vi "Register State as Status Example.vi"() -> ()   [LabVIEW 2017, in "Register State as Status Example.lvlib"]
uses:
  Register State as Status Example.lvlib
  user.lib/_NEVSTOP/Communicable State Machine(CSM)/Utility/_support/Periodic String Filter Level.ctl
  user.lib/_NEVSTOP/Communicable State Machine(CSM)/_Support/Common/Format Timestamp.vi
  user.lib/_NEVSTOP/Communicable State Machine(CSM)/AdvanceAPI/CSM - Revert Arguments-Safe String.vi
  user.lib/_NEVSTOP/Communicable State Machine(CSM)/AdvanceAPI/CSM - Make String Arguments Safe.vi
  user.lib/_NEVSTOP/Communicable State Machine(CSM)/AdvanceAPI/CSM - Break Down Multiple States String.vi
  user.lib/_NEVSTOP/Communicable State Machine(CSM)/AdvanceAPI/CSM - Compact Multiple States.vi
  user.lib/_NEVSTOP/Communicable State Machine(CSM)/AdvanceAPI/CSM - Keywords.vi
  user.lib/_NEVSTOP/Communicable State Machine(CSM)/_Shared/Trim Single-line Text.vi
  user.lib/_NEVSTOP/Communicable State Machine(CSM)/Communicable State Machine.lvlib
  user.lib/_NEVSTOP/Communicable State Machine(CSM)/Utility/Periodic String Filter Setting.ctl
  user.lib/_NEVSTOP/Communicable State Machine(CSM)/_Shared/CSM Shared.lvlib
panel:
  in  "Macro: Exit -> submodule2":bool
  in  "Macro: Exit -@submodule1":bool
  out "LogInQ":i32
  out "State History":string
  out "log handling Speed(#/s)":dbl
  out "LogInQ change(#/s)":dbl
  out "Level":T1
  in  "Registration":string="Macro: Initialize@* >> Echo: Echo1 -><register> \nAPI: API1@* >> Echo: Echo1-><register>\nAPI: API2@SubModule1 >> Echo: Echo2 -><register>\nEcho: Echo2@main >> API: API1@submodule1 -><register>\nExit@submodule1 >> Echo: Echo1 -><register>\nMacro: Exit@submodule2 >> Echo: Echo1 -><register>"
  in  "API: API2 -> submodule2":bool
  in  "API: API1 -> submodule2":bool
  in  "API: API2 -@submodule1":bool
  in  "API: API1 -@submodule1":bool
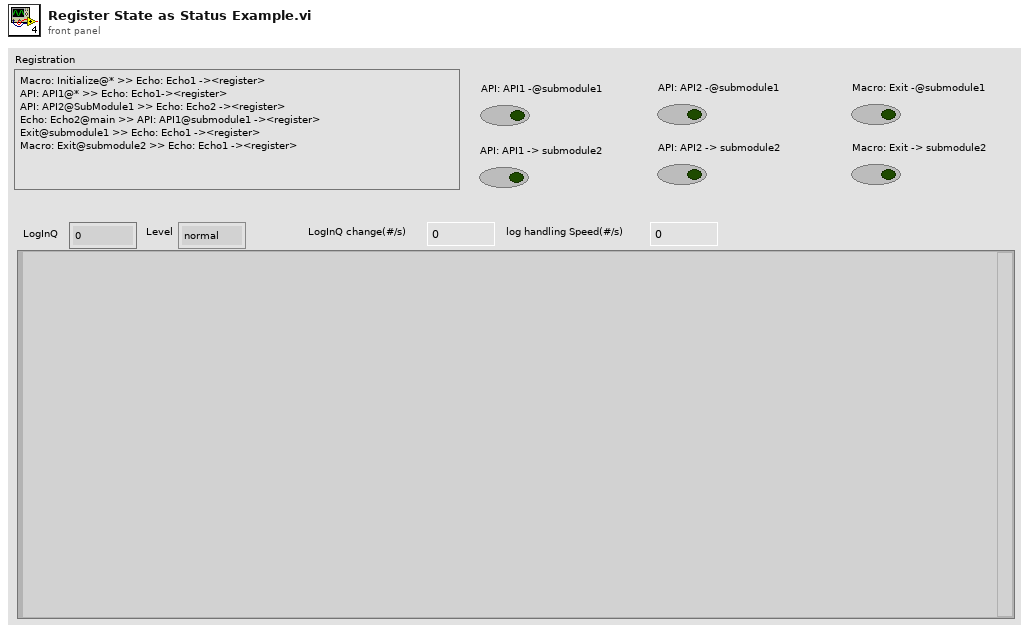
[diagram p1: front panel]
types:
  T1 = typedef "Communicable State Machine.lvlib/Periodic String Filter Level.ctl" = enum16{"normal", "L1", "L2", "L3", "L4"}
  T2 = enum32{"Invalid", "Standard", "Closed", "Hidden", "Minimized", "Maximized"}
  T3 = enum32{"invalid app kind", "Development System", "Run Time System", "Student Edition", "Embedded LabVIEW", "Evaluation", "Custom"}
  T4 = typedef "Communicable State Machine.lvlib/_CSM_Response Source Message.ctl" = cluster{"‘State":string, "’Arguments":string, "’Error":errorcluster}
  T5 = cluster{"Current VI Reference":refnum<vi>, "Close Panel on Exit?":bool}
  T6 = cluster{"Core":cluster{"Current VI Reference":refnum<vi>, "Close Panel on Exit?":bool}, "Your Boolean data":bool, "Your string data":string}
  T7 = typedef "Communicable State Machine.lvlib/_CSM_STATE_CALL_REASON.ctl" = enum16{"LocalCall", "RemoteCall", "StatusCallback"}
  T8 = typedef "Communicable State Machine.lvlib/Periodic String Filter Setting.ctl" = cluster{"threashold(#/s)":dbl, "Check Peroid(s)":dbl}
  T9 = typedef "Communicable State Machine.lvlib/_CSM_GlobalLog_MSG.ctl" = cluster{"Name (\"\" to Use UUID)":string, "Current State":string, "Arguments":string, "Source Message":T4, "Source Module":string, "Complete(T)/Start(F)":bool, "LogType":T10, "Time Stamp":timestamp}
  T10 = typedef "Communicable State Machine.lvlib/_CSM_GlobalLog_MSG_TYPE.ctl" = enum16{"User Log", "State Change", "Status", "Interrupt", "Register", "Unregister", "Error Log", "Module Created", "Module Destroyed"}
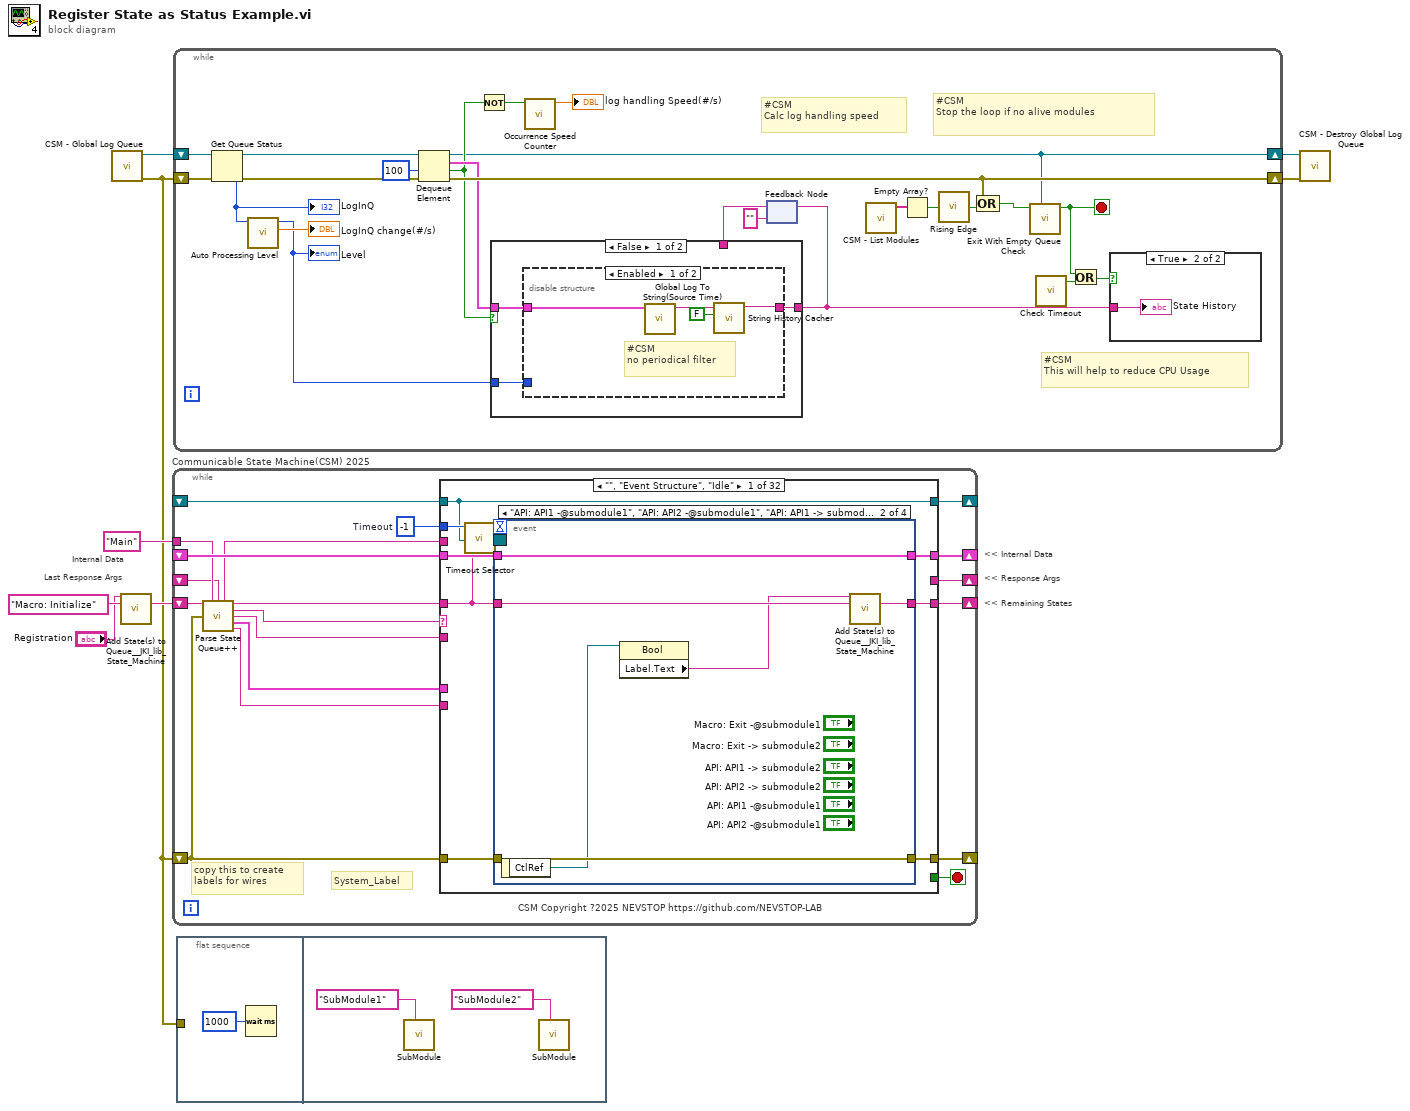
[diagram p0: block diagram]
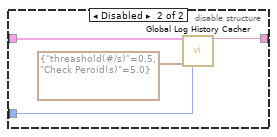
[diagram p2: hidden frame]
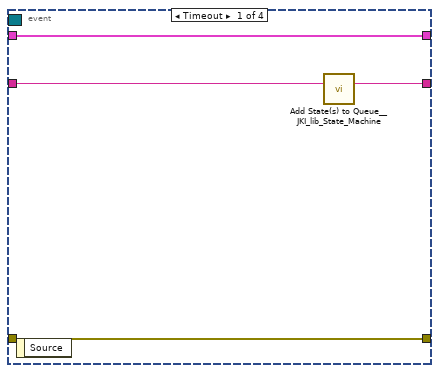
[diagram p5: hidden frame]
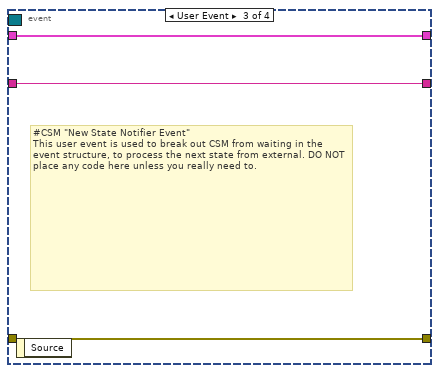
[diagram p6: hidden frame]
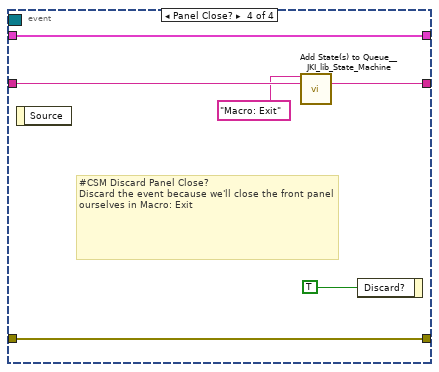
[diagram p7: hidden frame]
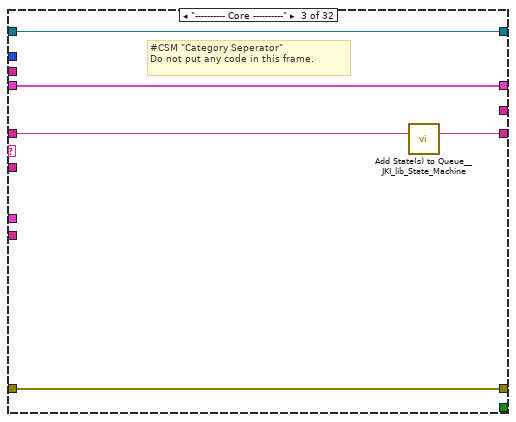
[diagram p9: hidden frame]
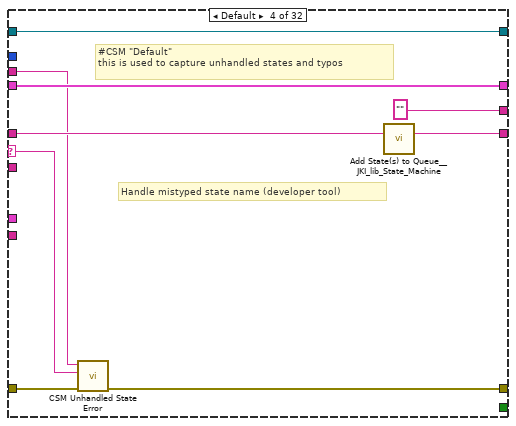
[diagram p10: hidden frame]
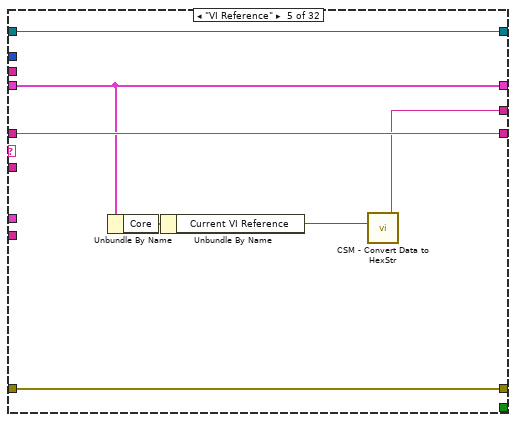
[diagram p11: hidden frame]
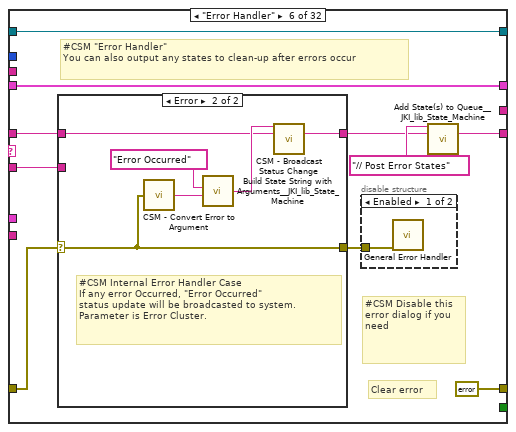
[diagram p12: hidden frame]
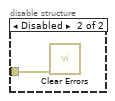
[diagram p13: hidden frame]
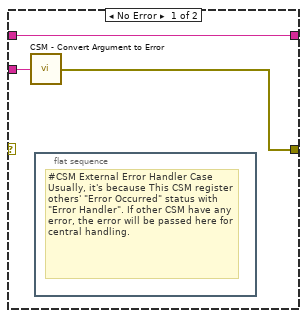
[diagram p14: hidden frame]
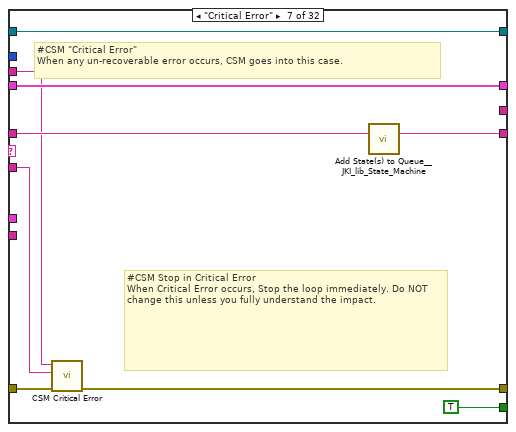
[diagram p15: hidden frame]
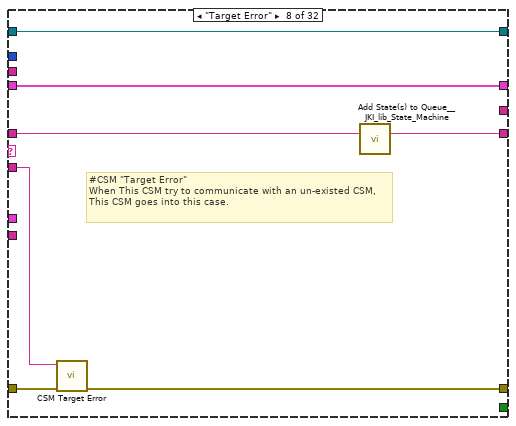
[diagram p16: hidden frame]
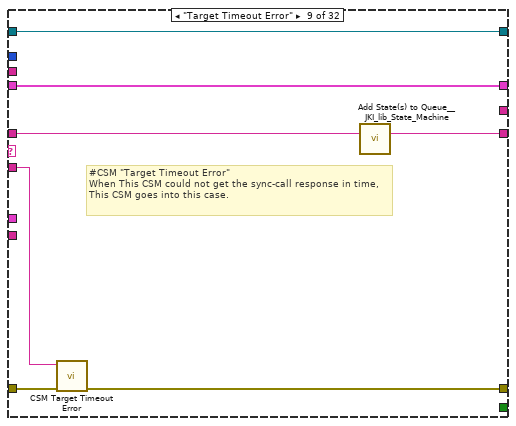
[diagram p17: hidden frame]
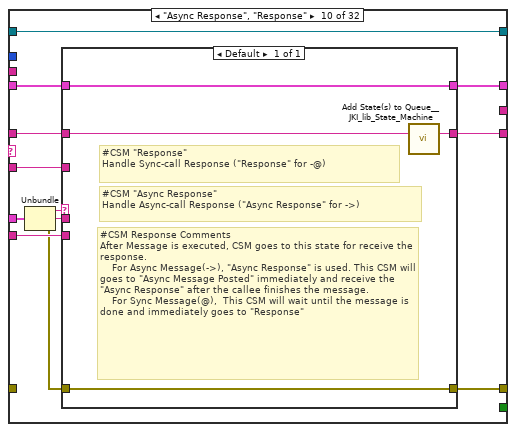
[diagram p18: hidden frame]
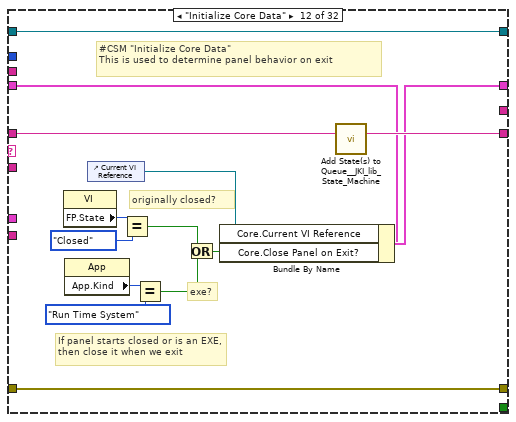
[diagram p20: hidden frame]
diagram:
  # "Last Response Args"
  # "Internal Data"
  # "<< Internal Data"
  # "<< Response Args"
  # "<< Remaining States"
  n1 = call "CSM - Global Log Queue.vi"() -> ("error out"=w1:errorcluster, "GlobalEvent Queue"=w2:refnum<queue>)  [unwired: 10 in]
  n2 = call <vilib>:"Add State(s) to Queue__JKI_lib_State_Machine.vi"("State(s) in Front (\"\")"="Registration", "State(s) in (\"\")"="Macro: Initialize" ("Init State(\"Macro: Initialize\")")) -> ("States Out"=w8:string)  [unwired: 13 in]
  n3 = while "Communicable State Machine(CSM) 2025" {
    shift-right: [w22] -> _
    shift-left: _ -> [w21]
    shift-right: [w25] -> _
    shift-left: w1 -> [w19]
    shift-right: [w24] -> _
    shift-left: w8 -> [w26]
    tunnel: "Main" ("Name(\"\" to use uuid)") -> [w15]
    shift-right: [w18] -> _
    shift-left: _ -> [w9]
    shift-right: [w17] -> _
    shift-left: _ -> [w16]
    stop <- w23 stop-if-true
    w20 = -1  # Timeout
    # "copy this to create labels for wires"
    # "System_Label"
    # "CSM Copyright ?2025 NEVSTOP https://github.com/NEVSTOP-LAB"
    n4 = call "Parse State Queue++.vi"("State Queue"=w26, "Name (\"\" to Use UUID)"=w15, "Response Arguments"=w9, "Previous Error"=w19) -> ("Name Used"=w10:string, "Remaining States"=w27:string, "Current State"=w14:string, "Arguments"=w13:string, ">> Response Source Message >>"=w12:T4, ">> Source CSM >>"=w11:string)  [unwired: 6 in]
    n5 = case shown="\"\", \"Event Structure\", \"Idle\"" w14 {
      selector: w14 -> [_ _ _ w67 _ _ _ _ _ _ _ _ _ _ _ _ _ _ _ _ _ _ _ _ _ _ _ _ _ _ _ _]
      tunnel: w27 -> [w28 w58 w64 w72 w79 w85 w108 w114 w121 w130 w143 w158 w164 w169 w177 w184 w189 w196 w200 w206 w211 w218 w234 w304 w310 w323 w326 w331 w337 w345 w355 w370]
      tunnel: w13 -> [_ _ _ _ _ w84 w103 w113 w120 w129 _ _ _ _ _ _ _ _ _ _ _ w213 w228 _ _ _ _ _ w334 _ w350 _]
      tunnel: w21 -> [w35 w57 w61 w70 w78 w89 w109 w116 w123 w132 w142 w151 w162 w166 _ w179 w186 w195 w199 w203 w209 w216 w230 w301 w307 w320 w325 w330 w336 w342 w352 w367]
      tunnel: [w34 w59 w62 w65 w80 errorcluster {"status"=FALSE, "code"=0, "source"=""} ("error out") w104 w111 w118 w135 w144 w155 w161 w167 w174 w180 w187 w190 w198 w204 w208 w214 w231 w302 w308 w321 w327 w332 w338 w343 w353 w368] -> w25
      tunnel: w19 -> [w33 w59 w62 w73 w80 w86 w110 w112 w119 _ w144 w155 w161 w167 w174 w181 w187 _ w201 w204 w208 w215 w232 w302 w308 w321 w327 w332 w338 w343 w353 w368]
      tunnel: [w36 w58 w63 w71 w79 w81 w107 w117 w124 w131 w143 w157 w163 w168 w176 w183 w188 w196 w200 w205 w210 w217 w233 w303 w309 w322 w326 w331 w337 w344 w354 w369] -> w24
      tunnel: [_ _ _ _ _ _ TRUE _ _ _ _ _ TRUE _ _ _ _ _ _ _ _ _ _ _ _ _ _ _ _ _ _ _] -> w23
      tunnel: [w32 w57 w61 w70 w78 w89 w109 w116 w123 w133 w142 w156 w162 w166 w175 w179 w186 w195 w199 w203 w209 w216 w230 w301 w307 w320 w325 w330 w336 w342 w352 w367] -> w22
      tunnel: w20 -> [w31 _ _ _ _ _ _ _ _ _ _ _ _ _ _ _ _ _ _ _ _ _ _ _ _ _ _ _ _ _ _ _]
      tunnel: w11 -> [_ _ _ _ _ _ _ _ _ w127 _ _ _ _ _ _ _ _ _ _ _ _ _ _ _ _ _ _ _ _ w348 _]
      tunnel: w12 -> [_ _ _ _ _ _ _ _ _ w134 _ _ _ _ _ _ _ _ _ _ _ _ _ _ _ _ _ _ _ _ w349 _]
      tunnel: [_ _ _ "" w74 _ _ _ _ _ _ _ _ _ _ _ _ _ _ _ _ _ _ _ _ _ _ "API1 Response" w333 _ _ _] -> w18
      tunnel: [w30 w56 w60 w68 w77 w88 w105 w115 w122 w136 w141 w145 w159 w165 w170 w178 w185 w194 w197 w202 w207 w212 w227 w300 w305 w313 w324 w329 w335 w341 w351 w366] -> w17
      tunnel: w16 -> [w30 w56 w60 w68 w77 w88 w105 w115 w122 w136 w141 w145 w159 w165 w170 w178 w185 _ w197 w202 w207 w212 w227 w300 w305 w313 w324 w329 w335 w341 w351 w366]
      tunnel: w10 -> [_ _ _ w66 _ _ w102 _ _ _ _ _ _ _ _ _ _ w193 _ _ _ _ _ _ _ _ _ _ _ _ _ _]
      frame "", "Event Structure", "Idle" {
        n6 = call "Timeout Selector.vi"("Remaining States"=w28, "Timeout Expected"=w31) -> ("Timeout"=w29:i32)  [unwired: 5 in]
        n7 = event shown="[1] \"API: API1 -@submodule1\", \"API: API2 -@submodule1\", \"API: API1 -> submodule2\", \"API: API2 -> submodule2\", \"Macro: Exit -@submodule1\", \"Macro: Exit -> submodule2\": Value Change" {
          selector: w30 -> [_ _ _ _]
          dyn-events: _ -> [_ _ _ _]
          timeout: w29 -> [_ _ _ _]
          tunnel: w28 -> [w40 w43 w48 w55]
          tunnel: [w39 w44 w48 w54] -> w36
          tunnel: w35 -> [w37 w45 w49 w52]
          tunnel: [w38 w46 w47 w53] -> w34
          tunnel: w33 -> [w38 w46 w47 w53]
          tunnel: [w37 w45 w49 w52] -> w32
          event Timeout {
            n8 = event-data() -> ()  [unwired: 1 in, 1 out]
            n9 = call <vilib>:"Add State(s) to Queue__JKI_lib_State_Machine.vi"("State(s) in (\"\")"=w40) -> ("States Out"=w39:string)  [unwired: 14 in]
          }
          event "API: API1 -@submodule1", "API: API2 -@submodule1", "API: API1 -> submodule2", "API: API2 -> submodule2", "Macro: Exit -@submodule1", "Macro: Exit -> submodule2": Value Change {
            n10 = event-data() -> ("CtlRef"=w42:refnum<vi>)  [unwired: 1 in]
            n11 = property class="Bool"(reference=w42) -> ("Label.Text"=w41:string)  [unwired: 1 in, 2 out]
            n12 = call <vilib>:"Add State(s) to Queue__JKI_lib_State_Machine.vi"("State(s) in Front (\"\")"=w41, "State(s) in (\"\")"=w43) -> ("States Out"=w44:string)  [unwired: 13 in]
          }
          event User Event {
            # "#CSM \"New State Notifier Event\"\nThis user event is used to break out CSM from waiting in the event structure, to process the next state from external. DO NOT place any code here unless you really need to."
            n13 = event-data() -> ()  [unwired: 1 in, 1 out]
          }
          event Panel Close? {
            # "#CSM Discard Panel Close?\nDiscard the event because we'll close the front panel ourselves in Macro: Exit"
            n14 = event-data() -> ()  [unwired: 1 in, 1 out]
            n15 = call <vilib>:"Add State(s) to Queue__JKI_lib_State_Machine.vi"("State(s) in Front (\"\")"="Macro: Exit", "State(s) in (\"\")"=w55) -> ("States Out"=w54:string)  [unwired: 13 in]
            n16 = event-data("Discard?"=TRUE) -> ()  [unwired: 1 in, 1 out]
          }
        }
      }
      frame "CSM Documentation" {
        # "#CSM README FIRST\n\nCommunicable State Machine(CSM) is a LabVIEW application framework that builds upon JKI State Machine(JKISM). It follows the pattern of JKISM and extends the keywords to describe message communication between modules, including concepts such as Sync-Message, Async-Message, Subscription/Unsubscription of status - essential elements for creating reusable code modules. For more information, please visit the CSM wiki: https://nevstop-lab.github.io/CSM-Wiki/\n\nFor instructions on JKI State Machine, visit: http://jki.net/state-machine/\nFor information about CSM, visit: https://github.com/NEVSTOP-LAB"
        # "#CSM \"Documentation\"\nCase for holding CSM Documenation"
      }
      frame "---------- Core ----------" {
        # "#CSM \"Category Seperator\"\nDo not put any code in this frame."
        n17 = call <vilib>:"Add State(s) to Queue__JKI_lib_State_Machine.vi"("State(s) in (\"\")"=w64) -> ("States Out"=w63:string)  [unwired: 14 in]
      }
      frame Default {
        # "#CSM \"Default\"\nthis is used to capture unhandled states and typos"
        # "Handle mistyped state name (developer tool)"
        n18 = call "CSM Unhandled State Error.vi"("error in (no error)"=w73, "Current State"=w67, "CSM Name"=w66) -> ("error out"=w65:errorcluster)  [unwired: 8 in]
        n19 = call <vilib>:"Add State(s) to Queue__JKI_lib_State_Machine.vi"("State(s) in (\"\")"=w72) -> ("States Out"=w71:string)  [unwired: 14 in]
      }
      frame "VI Reference" {
        n20 = Unbundle By Name(w78) -> ("Core"=w76:T5)
        n21 = Unbundle By Name(w76) -> ("Current VI Reference"=w75:refnum<vi>)
        n22 = call "CSM - Convert Data to HexStr.vi"("Variant"=w75) -> ("HEX String (0-9,A-F)"=w74:string)  [unwired: 8 in]
      }
      frame "Error Handler" {
        # "#CSM Disable this error dialog if you need"
        # "#CSM \"Error Handler\"\nYou can also output any states to clean-up after errors occur"
        # "Clear error"
        n23 = case shown="Error" w86 {
          selector: w86 -> [_ w96]
          tunnel: [w95 w98] -> w82
          tunnel: w85 -> [w95 w97]
          tunnel: w84 -> [w94 _]
          tunnel: [w93 w96] -> w87
          frame No Error {
            n24 = call "CSM - Convert Argument to Error.vi"("Argument"=w94) -> ("Error"=w93:errorcluster)  [unwired: 4 in]
            n25 = flat-sequence {
              frame #0 {
                # "#CSM External Error Handler Case\nUsually, it's because This CSM register others' \"Error Occurred\" status with \"Error Handler\". If other CSM have any error, the error will be passed here for central handling."
              }
            }
          }
          frame Error {
            # "#CSM Internal Error Handler Case \nIf any error Occurred, \"Error Occurred\" \nstatus update will be broadcasted to system.\nParameter is Error Cluster."
            n26 = call "CSM - Convert Error to Argument.vi"("Error"=w96) -> ("Argument"=w100:string)  [unwired: 4 in]
            n27 = call <vilib>:"Build State String with Arguments__JKI_lib_State_Machine.vi"("Arguments (\"\")"=w100, "State"="Error Occurred" ("Status with Arguments")) -> ("State with Arguments"=w99:string)  [unwired: 4 in]
            n28 = call "CSM - Broadcast Status Change.vi"("Status With Arguments"=w99, "State Queue"=w97) -> ("Remaining States"=w98:string)  [unwired: 13 in]
          }
        }
        n29 = disable-structure shown="Enabled" {
          disable-tunnel: w87 -> [w91 w92]
          frame Enabled {
            n30 = call <vilib>:"General Error Handler.vi"("error in (no error)"=w91) -> ()  [unwired: 10 in, 5 out]
          }
          frame Disabled {
            n31 = call <vilib>:"Clear Errors.vi"("error in (no error)"=w92) -> ()  [unwired: 5 in, 2 out]
          }
        }
        n32 = call <vilib>:"Add State(s) to Queue__JKI_lib_State_Machine.vi"("State(s) in Front (\"\")"="// Post Error States", "State(s) in (\"\")"=w82) -> ("States Out"=w81:string)  [unwired: 13 in]
      }
      frame "Critical Error" {
        # "#CSM Stop in Critical Error\nWhen Critical Error occurs, Stop the loop immediately. Do NOT change this unless you fully understand the impact."
        # "#CSM \"Critical Error\"\nWhen any un-recoverable error occurs, CSM goes into this case."
        n33 = call "CSM Critical Error.vi"("error in (no error)"=w110, "Arugments (As Reason)"=w103, "CSM Name"=w102) -> ("error out"=w104:errorcluster)  [unwired: 8 in]
        n34 = call <vilib>:"Add State(s) to Queue__JKI_lib_State_Machine.vi"("State(s) in (\"\")"=w108) -> ("States Out"=w107:string)  [unwired: 14 in]
      }
      frame "Target Error" {
        # "#CSM \"Target Error\"\nWhen This CSM try to communicate with an un-existed CSM, This CSM goes into this case."
        n35 = call "CSM Target Error.vi"("error in (no error)"=w112, "Arguments (As CSM Name)"=w113) -> ("error out"=w111:errorcluster)  [unwired: 9 in]
        n36 = call <vilib>:"Add State(s) to Queue__JKI_lib_State_Machine.vi"("State(s) in (\"\")"=w114) -> ("States Out"=w117:string)  [unwired: 14 in]
      }
      frame "Target Timeout Error" {
        # "#CSM \"Target Timeout Error\"\nWhen This CSM could not get the sync-call response in time, This CSM goes into this case."
        n37 = call "CSM Target Timeout Error.vi"("error in (no error)"=w119, "Arguments (As CSM Name)"=w120) -> ("error out"=w118:errorcluster)  [unwired: 9 in]
        n38 = call <vilib>:"Add State(s) to Queue__JKI_lib_State_Machine.vi"("State(s) in (\"\")"=w121) -> ("States Out"=w124:string)  [unwired: 14 in]
      }
      frame "Async Response", "Response" {
        n39 = Unbundle(w134) -> ("‘State"=w128:string, "’Arguments"=w126:string, "’Error"=w125:errorcluster)
        n40 = case shown="Default" w128 {
          tunnel: [w140] -> w135
          tunnel: w125 -> [w140]
          tunnel: [w139] -> w133
          tunnel: w132 -> [w139]
          tunnel: [w137] -> w131
          tunnel: w130 -> [w138]
          tunnel: w129 -> [_]
          tunnel: w127 -> [_]
          tunnel: w126 -> [_]
          frame Default {
            # "#CSM Response Comments\nAfter Message is executed, CSM goes to this state for receive the response.\n    For Async Message(->), \"Async Response\" is used. This CSM will goes to \"Async Message Posted\" immediately and receive the \"Async Response\" after the callee finishes the message.\n    For Sync Message(@),  This CSM will wait until the message is done and immediately goes to \"Response\""
            # "#CSM \"Async Response\"\nHandle Async-call Response (\"Async Response\" for ->)"
            # "#CSM \"Response\"\nHandle Sync-call Response (\"Response\" for -@)"
            n41 = call <vilib>:"Add State(s) to Queue__JKI_lib_State_Machine.vi"("State(s) in (\"\")"=w138) -> ("States Out"=w137:string)  [unwired: 14 in]
          }
        }
      }
      frame "Async Message Posted" {
        # "#CSM \"Async Message Posted\"\nAfter Async Message is posted (-> or ->| ), CSM goes to this state for post-action.\nYou can use Argument - State to tell which Async Message is called."
      }
      frame "Initialize Core Data" {
        # "#CSM \"Initialize Core Data\"\nThis is used to determine panel behavior on exit"
        # "originally closed?"
        # "exe?"
        # "If panel starts closed or is an EXE, then close it when we exit"
        n42 = property class="VI"() -> ("FP.State"=w148:T2)  [unwired: 2 in, 2 out]
        n43 = property class="App"() -> ("App.Kind"=w154:T3)  [unwired: 2 in, 2 out]
        n44 = control-ref of="Current VI Reference"() -> (w149:refnum<vi>)
        n45 = Equal?(x=w148, y=T2."Closed" ("Front Panel Window:State")) -> (x = y?=w146:bool)
        n46 = Equal?(x=w154, y=T3."Run Time System" ("Application:Kind")) -> (x = y?=w152:bool)
        n47 = Or(x=w146, y=w152) -> (x .or. y?=w150:bool)
        n48 = Bundle By Name(cluster=w151, "Core.Current VI Reference"=w149, "Core.Close Panel on Exit?"=w150) -> (w156:T6)
        n49 = call <vilib>:"Add State(s) to Queue__JKI_lib_State_Machine.vi"("State(s) in (\"\")"=w158) -> ("States Out"=w157:string)  [unwired: 14 in]
      }
      frame "Exit" {
        # "#CSM \"Exit\"\nCase for exiting the loop. No errors that occur here will be handled."
        n50 = call <vilib>:"Add State(s) to Queue__JKI_lib_State_Machine.vi"("State(s) in (\"\")"=w164) -> ("States Out"=w163:string)  [unwired: 14 in]
      }
      frame "---------- Data ----------" {
        # "#CSM \"Category Seperator\"\nDo not put any code in this frame."
        n51 = call <vilib>:"Add State(s) to Queue__JKI_lib_State_Machine.vi"("State(s) in (\"\")"=w169) -> ("States Out"=w168:string)  [unwired: 14 in]
      }
      frame "Data: Initialize" {
        w171 = T5 {"Current VI Reference"=refnum, "Close Panel on Exit?"=FALSE}  # Core
        w173 = TRUE  # Your Boolean data
        w172 = ""  # Your string data
        # "#CSM do not delete - used by framework"
        # "#CSM Expand Bundle to add new data elements to shift register data."
        # "#CSM Add new data here."
        # "Initialize the shift-register data, here.\n(data names are defined by what you wire into the bundle function)"
        n52 = Bundle("Core"=w171, "Your Boolean data"=w173, "Your string data"=w172) -> (w175:T6)  [unwired: 1 in]
        n53 = call <vilib>:"Add State(s) to Queue__JKI_lib_State_Machine.vi"("State(s) in (\"\")"=w177) -> ("States Out"=w176:string)  [unwired: 14 in]
      }
      frame "Data: Cleanup" {
        # "Cleanup any data and references, here.\n(this is called automatically, by the Macro: Exit)"
        n54 = Unbundle By Name(w179) -> ("Core.Current VI Reference"=w182:refnum<vi>)
        n55 = Close Reference(reference=w182, error in (no error)=w181) -> (error out=w180:errorcluster)
        n56 = call <vilib>:"Add State(s) to Queue__JKI_lib_State_Machine.vi"("State(s) in (\"\")"=w184) -> ("States Out"=w183:string)  [unwired: 14 in]
      }
      frame "---------- Events ----------" {
        # "#CSM \"Category Seperator\"\nDo not put any code in this frame."
        n57 = call <vilib>:"Add State(s) to Queue__JKI_lib_State_Machine.vi"("State(s) in (\"\")"=w189) -> ("States Out"=w188:string)  [unwired: 14 in]
      }
      frame "Events: Register" {
        # "#CSM \"Events: Register\"\nRegister user event. New Message Event is registered to break CSM waiting in event structure by default."
        # "#CSM Register New Message Event\nRegister message event to break Waiting in Event structure."
        n58 = call "CSM - Get New State Notifier Event.vi"("Name (\"\" to Use UUID) In"=w193) -> ("error out"=w191:errorcluster, "New State Notifier Event"=w192:refnum<user-event>)  [unwired: 9 in]
        n59 = register-events(error in=w191, w192) -> (reference out=w194:refnum<event-registration>, error out=w190:errorcluster)  [unwired: 1 in]
      }
      frame "Events: Unregister" {
        # "#CSM \"Events: Unregister\"\nUnregister user event."
        n60 = Unregister For Events(event registration refnum=w197, error in=w201) -> (error out=w198:errorcluster)
      }
      frame "---------- UI ----------" {
        # "#CSM \"Category Seperator\"\nDo not put any code in this frame."
        n61 = call <vilib>:"Add State(s) to Queue__JKI_lib_State_Machine.vi"("State(s) in (\"\")"=w206) -> ("States Out"=w205:string)  [unwired: 14 in]
      }
      frame "UI: Initialize" {
        # "#CSM \"UI: Initialize\"\nInitialize the User Interface, here.\n(this is called automatically, by the Macro: Init)"
        n62 = call <vilib>:"Add State(s) to Queue__JKI_lib_State_Machine.vi"("State(s) in (\"\")"=w211) -> ("States Out"=w210:string)  [unwired: 14 in]
      }
      frame "UI: Cursor Set" {
        # "#CSM \"UI: Cursor Set\"\nSet and Unset Cursor Busy.\n(Usage: \"UI: Cursor Set >> Busy|Idle\")"
        # "Argument"
        n63 = disable-structure shown="Default" {
          disable-tunnel: w215 -> [w221 w226]
          disable-tunnel: [w220 w226] -> w214
          disable-tunnel: w213 -> [w219 _]
          frame condition #0 (active) {
            n64 = case shown="\"Idle\", Default" w219 {
              tunnel: w221 -> [w223 w225]
              tunnel: [w222 w224] -> w220
              frame "Idle", Default {
                n65 = call <vilib>:"Unset Busy.vi"("error in (no error)"=w223) -> ("error out"=w222:errorcluster)  [unwired: 10 in]
              }
              frame "Busy" {
                n66 = call <vilib>:"Set Busy.vi"("error in (no error)"=w225) -> ("error out"=w224:errorcluster)  [unwired: 9 in, 1 out]
              }
            }
          }
          frame condition #1 {
          }
        }
        n67 = call <vilib>:"Add State(s) to Queue__JKI_lib_State_Machine.vi"("State(s) in (\"\")"=w218) -> ("States Out"=w217:string)  [unwired: 14 in]
      }
      frame "UI: Front Panel State" {
        # "#CSM \"UI: Front Panel State\"\nSet Front Panel Open or Closed\n(Usage: \"UI: Front Panel State >> Open|Close\")"
        # "Argument"
        n68 = Unbundle By Name(w230) -> ("Core.Current VI Reference"=w229:refnum<vi>)
        n69 = call <vilib>:"Add State(s) to Queue__JKI_lib_State_Machine.vi"("State(s) in (\"\")"=w234) -> ("States Out"=w233:string)  [unwired: 14 in]
        n70 = case shown="\"Close\", \"Closed\"" w228 {
          tunnel: w232 -> [w240 w255 w266 w279 w292]
          tunnel: [w242 w256 w268 w281 w294] -> w231
          tunnel: w229 -> [w241 w253 w267 w280 w293]
          frame "Open", "Standard", Default {
            w235 = T2."Standard" ("State")
            n71 = property class="VI"(reference=w241, error in=w240) -> (reference out=w238:refnum<vi>, error out=w239:errorcluster, "FP.State"=w237:T2)
            n72 = Not Equal?(x=w237, y=w235) -> (x != y?=w236:bool)
            n73 = case shown="True" w236 {
              tunnel: [w246 w248] -> w242
              tunnel: w239 -> [w245 w248]
              tunnel: w238 -> [w244 _]
              tunnel: w235 -> [w243 _]
              frame True {
                n74 = invoke class="VI" method="FP.Open"(reference=w244, error in=w245, "Activate"=TRUE, "State"=w243) -> (error out=w246:errorcluster)  [unwired: 1 in, 4 out]
              }
              frame False {
              }
            }
          }
          frame "Close", "Closed" {
            n75 = property class="VI"(reference=w253, error in=w255) -> (reference out=w252:refnum<vi>, error out=w254:errorcluster, "FP.State"=w250:T2)
            n76 = Not Equal?(x=w250, y=T2."Closed" ("Front Panel Window:State")) -> (x != y?=w249:bool)
            n77 = case shown="False" w249 {
              tunnel: [w257 w260] -> w256
              tunnel: w254 -> [w257 w259]
              tunnel: w252 -> [_ w258]
              frame False {
              }
              frame True {
                n78 = invoke class="VI" method="FP.Close"(reference=w258, error in=w259) -> (error out=w260:errorcluster)  [unwired: 1 in, 2 out]
              }
            }
          }
          frame "Hidden", "Hide" {
            w261 = T2."Hidden" ("State")
            n79 = property class="VI"(reference=w267, error in=w266) -> (reference out=w264:refnum<vi>, error out=w265:errorcluster, "FP.State"=w263:T2)
            n80 = Not Equal?(x=w263, y=w261) -> (x != y?=w262:bool)
            n81 = case shown="True" w262 {
              tunnel: [w272 w273] -> w268
              tunnel: w265 -> [w271 w273]
              tunnel: w264 -> [w270 _]
              tunnel: w261 -> [w269 _]
              frame True {
                n82 = invoke class="VI" method="FP.Open"(reference=w270, error in=w271, "State"=w269) -> (error out=w272:errorcluster)  [unwired: 2 in, 4 out]
              }
              frame False {
              }
            }
          }
          frame "Minimize", "Minimized" {
            w274 = T2."Minimized" ("State")
            n83 = property class="VI"(reference=w280, error in=w279) -> (reference out=w277:refnum<vi>, error out=w278:errorcluster, "FP.State"=w276:T2)
            n84 = Not Equal?(x=w276, y=w274) -> (x != y?=w275:bool)
            n85 = case shown="True" w275 {
              tunnel: [w285 w286] -> w281
              tunnel: w278 -> [w284 w286]
              tunnel: w277 -> [w283 _]
              tunnel: w274 -> [w282 _]
              frame True {
                n86 = invoke class="VI" method="FP.Open"(reference=w283, error in=w284, "State"=w282) -> (error out=w285:errorcluster)  [unwired: 2 in, 4 out]
              }
              frame False {
              }
            }
          }
          frame "Maximize", "Maximized" {
            w287 = T2."Maximized" ("State")
            n87 = property class="VI"(reference=w293, error in=w292) -> (reference out=w290:refnum<vi>, error out=w291:errorcluster, "FP.State"=w289:T2)
            n88 = Not Equal?(x=w289, y=w287) -> (x != y?=w288:bool)
            n89 = case shown="True" w288 {
              tunnel: [w298 w299] -> w294
              tunnel: w291 -> [w297 w299]
              tunnel: w290 -> [w296 _]
              tunnel: w287 -> [w295 _]
              frame True {
                n90 = invoke class="VI" method="FP.Open"(reference=w296, error in=w297, "State"=w295) -> (error out=w298:errorcluster)  [unwired: 2 in, 4 out]
              }
              frame False {
              }
            }
          }
        }
      }
      frame "---------- Macro ----------" {
        # "#CSM \"Category Seperator\"\nDo not put any code in this frame."
        n91 = call <vilib>:"Add State(s) to Queue__JKI_lib_State_Machine.vi"("State(s) in (\"\")"=w304) -> ("States Out"=w303:string)  [unwired: 14 in]
      }
      frame "Macro: Initialize" {
        w306 = "Data: Initialize\nInitialize Core Data\nEvents: Register\nUI: Initialize\nUI: Front Panel State >> Open"  # Data: Initialize Initialize Core Data Events: Register UI: Initialize UI: Front Panel State >> Open
        # "#CSM \"Macro: Initialize\"\nInitialization Macro (This is called once, when the VI starts)"
        n92 = call <vilib>:"Add State(s) to Queue__JKI_lib_State_Machine.vi"("State(s) in Front (\"\")"=w306, "State(s) in (\"\")"=w310) -> ("States Out"=w309:string)  [unwired: 13 in]
      }
      frame "Macro: Exit" {
        # "#CSM \"Macro: Exit\"\nExit Macro (This is called once, when the VI exits)"
        n93 = Unbundle By Name(w320) -> ("Core.Close Panel on Exit?"=w319:bool)
        n94 = Select(t="UI: Front Panel State >> Close", s=w319, f="") -> (s? t:f=w316:string)
        n95 = call "CSM - Filter Messages to Non-Existing Modules.vi"("State (S) In (\"\")"="//Exit Sub-Modules \nMacro: Exit -@ Submodule1\nMacro: Exit -@ Submodule2") -> ("States Out"=w311:string)  [unwired: 14 in]
        n96 = call <vilib>:"Add State(s) to Queue__JKI_lib_State_Machine.vi"("State(s) in Front (\"\")"=w311, "State(s) in (\"\")"=w316, "State(s) at Back (\"\")"="Data: Cleanup\nEvents: Unregister\nExit") -> ("States Out"=w314:string)  [unwired: 12 in]
        n97 = call <vilib>:"Add State(s) to Queue__JKI_lib_State_Machine.vi"("State(s) in Front (\"\")"=w314, "State(s) in (\"\")"=w323) -> ("States Out"=w322:string)  [unwired: 13 in]
      }
      frame "---------- API ----------" {
        # "#CSM \"Category Seperator\"\nDo not put any code in this frame."
      }
      frame "API: API1" {
        # "#CSM API Example\nCopy/Rename this case for your own API"
        # "#CSM Response\nConnect this to return the response of your API"
        # "#CSM >> Source CSM >>\nIf you need to tell who triggered this state , use this string. If it's this case itself, this string is \"\"."
        # "#CSM >> Arguments >>\nDeal with the parameter if any"
      }
      frame "API: API2" {
        # "#CSM API Example\nCopy/Rename this case for your own API"
        # "unpack Hex String  to Variant\nif complex parameter is needed."
        n98 = call "CSM - Convert HexStr to Data.vi"("HEX String"=w334) -> ()  [unwired: 7 in, 2 out]
        n99 = disable-structure shown="Disabled" {
          disable-tunnel: [w339 "API2 Response"] -> w333
          frame Disabled {
            # "pack variant to hexstr \nif complex response is needed."
            # "complex Response"
            n100 = call "CSM - Convert Data to HexStr.vi"() -> ("HEX String (0-9,A-F)"=w339:string)  [unwired: 9 in]
          }
          frame Enabled {
          }
        }
      }
      frame "---------- Action ----------" {
        # "#CSM \"Category Seperator\"\nDo not put any code in this frame."
        n101 = call <vilib>:"Add State(s) to Queue__JKI_lib_State_Machine.vi"("State(s) in (\"\")"=w345) -> ("States Out"=w344:string)  [unwired: 14 in]
      }
      frame "Echo: Echo1" {
        # "#CSM \"Internal State\"\nThis category is used for holding internal states"
        n102 = call "State Triggered Reason.vi"(">> Source CSM >> (In)"=w348, ">> Response Source Message >> (In)"=w349) -> ("Reason"=w347:T7, ">> Response Source Message >>"=w346:T4)  [unwired: 7 in, 1 out]
        n103 = case shown="\"StatusCallback\"" w347 {
          selector: w347 -> [_ w359]
          tunnel: w350 -> [_ w361]
          tunnel: w348 -> [_ w362]
          tunnel: w346 -> [_ w364]
          frame Default {
          }
          frame "StatusCallback" {
            n104 = Unbundle By Name(w364) -> ("‘State"=w363:string, "’Error"=w357:errorcluster)
            n105 = call "CSM - Convert Error to Argument.vi"("Error"=w357) -> ("Argument"=w356:string)  [unwired: 4 in]
            n106 = Format Into String(format string="\"%s\" from \"%s\"\nResponse: \"%s\"\nerror: \"%s\"", w363, w362, w361, w356) -> (resulting string=w360:string)  [unwired: 2 in, 1 out]
            n107 = Format Into String(w359) -> (resulting string=w358:string)  [unwired: 3 in, 1 out]
            n108 = One Button Dialog(message=w360, button name ("OK")=w358) -> ()  [unwired: 1 out]
          }
        }
        n109 = call <vilib>:"Add State(s) to Queue__JKI_lib_State_Machine.vi"("State(s) in (\"\")"=w355) -> ("States Out"=w354:string)  [unwired: 14 in]
      }
      frame "Echo: Echo2" {
        # "#CSM \"Internal State\"\nThis category is used for holding internal states"
        n110 = call <vilib>:"Add State(s) to Queue__JKI_lib_State_Machine.vi"("State(s) in (\"\")"=w370) -> ("States Out"=w369:string)  [unwired: 14 in]
      }
    }
  }
  n111 = while {
    shift-right: [w393] -> w4
    shift-left: w1 -> [w390]
    shift-right: [w377] -> w3
    shift-left: w2 -> [w394]
    stop <- w371 stop-if-true
    # "#CSM\nCalc log handling speed"
    # "#CSM\nStop the loop if no alive modules"
    # "#CSM\nThis will help to reduce CPU Usage"
    n112 = Get Queue Status(queue=w394, error in (no error)=w390) -> (queue out=w392:refnum<queue>, error out=w391:errorcluster, # elements in queue=w373:i32)  [unwired: 1 in, 5 out]
    "LogInQ" <- w373
    n113 = call "Auto Processing Level.vi"("#Left In Q"=w373) -> ("LogInQ Changing Speed (#/s)"=→"LogInQ change(#/s)":dbl, "Level"=w372:T1)  [unwired: 8 in, 1 out]
    "Level" <- w372
    n114 = Dequeue Element(queue=w392, timeout in ms (-1)=100, error in (no error)=w391) -> (queue out=w377:refnum<queue>, element=w389:T9, timed out?=w379:bool, error out=w393:errorcluster)
    n115 = Not(x=w379) -> (.not. x?=w378:bool)
    n116 = call "Occurrence Speed Counter.vi"("Occured? (T)"=w378) -> ("Speed (#/s)"=→"log handling Speed(#/s)":dbl)  [unwired: 8 in, 2 out]
    n117 = feedback #1("" ("String Cache")) -> (w385:string)
    n118 = case shown="False" w379 {
      tunnel: w389 -> [w397 _]
      tunnel: [w396 w406] -> w386
      tunnel: w385 -> [_ w406]
      tunnel: w372 -> [w395 _]
      frame False {
        n119 = disable-structure shown="Enabled" {
          disable-tunnel: w397 -> [w401 w404]
          disable-tunnel: [w399 w405] -> w396
          disable-tunnel: w395 -> [_ w403]
          frame Enabled {
            # "#CSM \nno periodical filter"
            n120 = call "Global Log To String(Source Time).vi"("Log"=w401) -> ("Log String"=w400:string)  [unwired: 9 in]
            n121 = call "String History Cacher.vi"("Include Timestamp? (T)"=FALSE ("Include Timestamp(T)"), "String"=w400) -> ("String Cache"=w399:string)  [unwired: 9 in]
          }
          frame Disabled {
            n122 = call "Global Log History Cacher.vi"("Cross CSM Data"=w404, "Settings"=T8 {"threashold(#/s)"=0.5, "Check Peroid(s)"=5.0}, "Level (Normal)"=w403) -> ("String Cache"=w405:string)  [unwired: 12 in]
          }
        }
      }
      frame True {
      }
    }
    n123 = feedback-in #1(w386) -> ()
    n124 = call "CSM - List Modules.vi"() -> ("Module Names"=w384:string[])  [unwired: 10 in, 1 out]
    n125 = Empty Array?(array=w384) -> (empty?=w383:bool)
    n126 = call "Rising Edge.vi"("Signal"=w383) -> ("Rising Edge"=w382:bool)
    n127 = Compound Arithmetic op=OR(w393, w382) -> (w375:bool)
    n128 = call "Exit With Empty Queue Check.vi"("Queue"=w377, "Stop"=w375) -> ("Exit"=w371:bool)  [unwired: 8 in, 1 out]
    n129 = call "Check Timeout.vi"() -> ("Timeout"=w387:bool)  [unwired: 8 in]
    n130 = Or(x=w371, y=w387) -> (x .or. y?=w376:bool)
    n131 = case shown="True" w376 {
      tunnel: w386 -> [_ w407]
      frame False {
      }
      frame True {
        "State History" <- w407
      }
    }
  }
  n132 = flat-sequence {
    tunnel: w1 -> [_]
    frame #0 {
      n133 = Wait (ms)(milliseconds to wait=u32 1000) -> ()  [unwired: 1 out]
    }
    frame #1 {
      n134 = call "SubModule.vi"("Name (\"\" to Use Uuid)"="SubModule1" ("Name(\"\" to use uuid)")) -> ()  [unwired: 11 in]
      n135 = call "SubModule.vi"("Name (\"\" to Use Uuid)"="SubModule2" ("Name(\"\" to use uuid)")) -> ()  [unwired: 11 in]
    }
  }
  n136 = call "CSM - Destroy Global Log Queue.vi"("Error In"=w4, "Global Log Queue"=w3) -> ()  [unwired: 9 in, 1 out]
